vi "Lab Panel V5.26.vi"() -> ()   [LabVIEW 2017] (continued)
                    n1483 = Unbundle(w2774) -> ("T-RISE mins"=w2773:dbl)  [unwired: 4 out]
                    n1484 = Greater Or Equal?(x=w2776, y=w2775) -> (x >= y?=w2777:bool)
                    n1485 = case shown="True" w2777 {
                      tunnel: w2773 -> [w2780 _]
                      tunnel: w2772 -> [w2779 _]
                      tunnel: w2771 -> [w2778 _]
                      frame True {
                        n1486 = stacked-sequence {
                          tunnel: w2780 -> [w2783 _]
                          tunnel: w2779 -> [_ w2788]
                          tunnel: w2778 -> [w2781 _]
                          frame #0 {
                            n1487 = Build Array("T-RISE") -> (w2785:string[])
                            n1488 = Build Array(w2783) -> (w2784:dbl[])
                            n1489 = TDMS Write(0:w2781, 5:"TEST PASS", 7:w2785, 9:w2784) -> (15:w2787:errorcluster)  [unwired: 2 in, 3 out]
                            n1490 = local write "data file error"(w2787) -> ()
                          }
                          frame #1 {
                            n1491 = Bundle(cluster=w2788, "STATUS"="T-RISE PASS") -> (w2790:T4)  [unwired: 2 in]
                            n1492 = local write "RESULT LAB04-2"(TRUE) -> ()
                            n1493 = local write "DISP LAB04-2"(w2790) -> ()
                          }
                        }
                      }
                      frame False {
                      }
                    }
                  }
                }
              }
              frame #8 {
                # "LAB05-1"
                n1494 = Equal?(x=w2793, y=2) -> (x = y?=w2796:bool)
                n1495 = local read "DISP LAB05-1"() -> (w2798:T4)
                n1496 = Unbundle(w2798) -> ("STATUS"=w2799:string)  [unwired: 2 out]
                n1497 = Equal?(x=w2799, y="RUN") -> (x = y?=w2795:bool)
                n1498 = And(x=w2795, y=w2796) -> (x .and. y?=w2794:bool)
                n1499 = case shown="True" w2794 {
                  tunnel: w2798 -> [_ w2802]
                  tunnel: w2792 -> [_ w2805]
                  frame False {
                  }
                  frame True {
                    n1500 = local read "SET LAB05-1"() -> (w2804:T5)
                    n1501 = local read "TDMS LAB05-1"() -> (w2801:refnum<k34>)
                    n1502 = Unbundle(w2802) -> ("CYCLE"=w2806:dbl)  [unwired: 2 out]
                    n1503 = Unbundle(w2804) -> ("T-RISE mins"=w2803:dbl)  [unwired: 4 out]
                    n1504 = Greater Or Equal?(x=w2806, y=w2805) -> (x >= y?=w2807:bool)
                    n1505 = case shown="True" w2807 {
                      tunnel: w2803 -> [w2810 _]
                      tunnel: w2802 -> [w2809 _]
                      tunnel: w2801 -> [w2808 _]
                      frame True {
                        n1506 = stacked-sequence {
                          tunnel: w2810 -> [w2813 _]
                          tunnel: w2809 -> [_ w2818]
                          tunnel: w2808 -> [w2811 _]
                          frame #0 {
                            n1507 = Build Array("T-RISE") -> (w2815:string[])
                            n1508 = Build Array(w2813) -> (w2814:dbl[])
                            n1509 = TDMS Write(0:w2811, 5:"TEST PASS", 7:w2815, 9:w2814) -> (15:w2817:errorcluster)  [unwired: 2 in, 3 out]
                            n1510 = local write "data file error"(w2817) -> ()
                          }
                          frame #1 {
                            n1511 = Bundle(cluster=w2818, "STATUS"="T-RISE PASS") -> (w2820:T4)  [unwired: 2 in]
                            n1512 = local write "RESULT LAB05-1"(TRUE) -> ()
                            n1513 = local write "DISP LAB05-1"(w2820) -> ()
                          }
                        }
                      }
                      frame False {
                      }
                    }
                  }
                }
              }
              frame #9 {
                # "LAB05-2"
                n1514 = Equal?(x=w2823, y=2) -> (x = y?=w2826:bool)
                n1515 = local read "DISP LAB05-2"() -> (w2828:T4)
                n1516 = Unbundle(w2828) -> ("STATUS"=w2829:string)  [unwired: 2 out]
                n1517 = Equal?(x=w2829, y="RUN") -> (x = y?=w2825:bool)
                n1518 = And(x=w2825, y=w2826) -> (x .and. y?=w2824:bool)
                n1519 = case shown="True" w2824 {
                  tunnel: w2828 -> [_ w2832]
                  tunnel: w2822 -> [_ w2835]
                  frame False {
                  }
                  frame True {
                    n1520 = local read "SET LAB05-2"() -> (w2834:T5)
                    n1521 = local read "TDMS LAB05-2"() -> (w2831:refnum<k34>)
                    n1522 = Unbundle(w2832) -> ("CYCLE"=w2836:dbl)  [unwired: 2 out]
                    n1523 = Unbundle(w2834) -> ("T-RISE mins"=w2833:dbl)  [unwired: 4 out]
                    n1524 = Greater Or Equal?(x=w2836, y=w2835) -> (x >= y?=w2837:bool)
                    n1525 = case shown="True" w2837 {
                      tunnel: w2833 -> [w2840 _]
                      tunnel: w2832 -> [w2839 _]
                      tunnel: w2831 -> [w2838 _]
                      frame True {
                        n1526 = stacked-sequence {
                          tunnel: w2840 -> [w2843 _]
                          tunnel: w2839 -> [_ w2848]
                          tunnel: w2838 -> [w2841 _]
                          frame #0 {
                            n1527 = Build Array("T-RISE") -> (w2845:string[])
                            n1528 = Build Array(w2843) -> (w2844:dbl[])
                            n1529 = TDMS Write(0:w2841, 5:"TEST PASS", 7:w2845, 9:w2844) -> (15:w2847:errorcluster)  [unwired: 2 in, 3 out]
                            n1530 = local write "data file error"(w2847) -> ()
                          }
                          frame #1 {
                            n1531 = Bundle(cluster=w2848, "STATUS"="T-RISE PASS") -> (w2850:T4)  [unwired: 2 in]
                            n1532 = local write "RESULT LAB05-2"(TRUE) -> ()
                            n1533 = local write "DISP LAB05-2"(w2850) -> ()
                          }
                        }
                      }
                      frame False {
                      }
                    }
                  }
                }
              }
            }
          }
          frame #7 {
            # "end test & close test files"
            n1534 = local read "MAIL SETTINGS"() -> (w2856:T7)
            n1535 = Unbundle(w2856) -> ("OUT SERVER ADDRESS"=w2855:string, "FROM ACCOUNT"=w2854:string)  [unwired: 5 out]
            n1536 = stacked-sequence {
              tunnel: w2866 -> [_ _ _ _ _ _ _ _ _ _]
              tunnel: w2867 -> [_ _ _ _ _ _ _ _ _ _]
              tunnel: w2865 -> [_ _ _ _ _ _ _ _ _ _]
              tunnel: w2864 -> [_ _ _ _ _ _ _ _ _ _]
              tunnel: w2863 -> [_ _ _ _ _ _ _ _ _ _]
              tunnel: w2862 -> [_ _ _ _ _ _ _ _ _ _]
              tunnel: w2861 -> [_ _ _ _ _ _ _ _ _ _]
              tunnel: w2860 -> [_ _ _ _ _ _ _ _ _ _]
              tunnel: w2859 -> [_ _ _ _ _ _ _ _ _ _]
              tunnel: w2858 -> [_ _ _ _ _ _ _ _ _ _]
              tunnel: w2855 -> [w2871 w2923 w2971 w3018 w3065 w3112 w3159 w3206 w3253 w3300]
              tunnel: w2854 -> [w2870 w2922 w2970 w3017 w3064 w3111 w3158 w3205 w3252 w3299]
              tunnel: "Mail Test File To:" -> [w2869 w2921 w2969 w3016 w3063 w3110 w3157 w3204 w3251 w3298]
              tunnel: "Mail Test Fail" -> [w2868 w2920 w2968 w3015 w3062 w3109 w3156 w3203 w3250 w3297]
              frame #0 {
                # "LAB01-1"
                n1537 = local read "DISP LAB01-1"() -> (w2875:T4)
                n1538 = local read "run lab01-1"() -> (w2872:bool)
                n1539 = local read "TDMS LAB01-1"() -> (w2873:refnum<k34>)
                n1540 = Unbundle(w2875) -> ("CYCLE"=w2876:dbl, "STATUS"=w2874:string)  [unwired: 1 out]
                n1541 = case shown="True" w2872 {
                  tunnel: w2876 -> [_ w2882]
                  tunnel: w2875 -> [_ w2884]
                  tunnel: w2874 -> [_ w2881]
                  tunnel: w2873 -> [_ w2883]
                  tunnel: w2871 -> [_ w2880]
                  tunnel: w2870 -> [_ w2879]
                  tunnel: w2869 -> [_ w2878]
                  tunnel: w2868 -> [_ w2877]
                  frame False {
                  }
                  frame True {
                    n1542 = Not Equal?(x=w2881, y="RUN") -> (x != y?=w2885:bool)
                    n1543 = Greater?(x=w2882, y=2.0) -> (0:w2887:bool)
                    n1544 = And(x=w2887, y=w2885) -> (x .and. y?=w2886:bool)
                    n1545 = case shown="True" w2886 {
                      tunnel: w2884 -> [_ w2897]
                      tunnel: w2883 -> [_ w2896]
                      tunnel: w2882 -> [_ w2895]
                      tunnel: w2881 -> [_ w2894]
                      tunnel: w2880 -> [_ w2893]
                      tunnel: w2879 -> [_ w2892]
                      tunnel: w2878 -> [_ w2891]
                      tunnel: w2877 -> [_ w2890]
                      frame False {
                      }
                      frame True {
                        n1546 = stacked-sequence {
                          tunnel: w2897 -> [w2901 _ _]
                          tunnel: w2896 -> [_ w2903 _]
                          tunnel: w2895 -> [_ _ _]
                          tunnel: w2894 -> [_ _ w2909]
                          tunnel: w2893 -> [_ _ w2908]
                          tunnel: w2892 -> [_ _ w2907]
                          tunnel: w2891 -> [_ _ w2906]
                          tunnel: w2890 -> [_ _ w2905]
                          frame #0 {
                            w2898 = FALSE
                            n1547 = local write "mail control"("END") -> ()
                            n1548 = Bundle(cluster=w2901) -> (w2900:T4)  [unwired: 3 in]
                            n1549 = local write "DISP LAB01-1"(w2900) -> ()
                            n1550 = local write "O/I  LAB01-1"(w2898) -> ()
                            n1551 = local write "run lab01-1"(w2898) -> ()
                            n1552 = local write "RUN LAB01-1"(w2898) -> ()
                          }
                          frame #1 {
                            n1553 = TDMS Close(11:w2903) -> (0:w2902:errorcluster)  [unwired: 1 in, 1 out]
                            n1554 = local write "data file error"(w2902) -> ()
                          }
                          frame #2 {
                            n1555 = stacked-sequence {
                              tunnel: "LAB01-1" -> [w2911 w2913 _]
                              tunnel: w2909 -> [_ w2919 _]
                              tunnel: w2908 -> [_ w2918 _]
                              tunnel: w2907 -> [_ w2917 _]
                              tunnel: w2906 -> [_ w2916 _]
                              tunnel: w2905 -> [_ w2915 _]
                              frame #0 {
                                n1556 = call "sub vi - defrag tdms v1.vi"("panel id"=w2911) -> ("error out"=w2910:errorcluster)  [unwired: 10 in]
                                n1557 = local write "data file error"(w2910) -> ()
                              }
                              frame #1 {
                                n1558 = Bundle("STATUS"=w2919, "OUT SERVER ADDRESS"=w2918, "FROM ACCOUNT"=w2917, "Mail Test File To:"=w2916, "Mail Test Fail"=w2915) -> (w2912:T26)  [unwired: 1 in]
                                n1559 = call "Save data file (pass-fail) v5.vi"("Input Cluster"=w2912, "panel id"=w2913) -> ("network file save error"=w2914:errorcluster)  [unwired: 8 in, 1 out]
                                n1560 = local write "data file error"(w2914) -> ()
                              }
                              frame #2 {
                              }
                            }
                          }
                        }
                      }
                    }
                  }
                }
              }
              frame #1 {
                # "LAB01-2"
                n1561 = local read "run lab01-2"() -> (w2924:bool)
                n1562 = case shown="True" w2924 {
                  tunnel: w2923 -> [_ w2928]
                  tunnel: w2922 -> [_ w2927]
                  tunnel: w2921 -> [_ w2926]
                  tunnel: w2920 -> [_ w2925]
                  frame False {
                  }
                  frame True {
                    n1563 = local read "DISP LAB01-2"() -> (w2936:T4)
                    n1564 = local read "TDMS LAB01-2"() -> (w2935:refnum<k34>)
                    n1565 = Unbundle(w2936) -> ("CYCLE"=w2930:dbl, "STATUS"=w2929:string)  [unwired: 1 out]
                    n1566 = Not Equal?(x=w2929, y="RUN") -> (x != y?=w2932:bool)
                    n1567 = Greater?(x=w2930, y=2.0) -> (0:w2933:bool)
                    n1568 = And(x=w2933, y=w2932) -> (x .and. y?=w2931:bool)
                    n1569 = case shown="True" w2931 {
                      tunnel: w2936 -> [_ w2945]
                      tunnel: w2935 -> [_ w2944]
                      tunnel: w2930 -> [_ w2943]
                      tunnel: w2929 -> [_ w2942]
                      tunnel: w2928 -> [_ w2941]
                      tunnel: w2927 -> [_ w2940]
                      tunnel: w2926 -> [_ w2939]
                      tunnel: w2925 -> [_ w2938]
                      frame False {
                      }
                      frame True {
                        n1570 = stacked-sequence {
                          tunnel: w2945 -> [w2948 _ _]
                          tunnel: w2944 -> [_ w2950 _]
                          tunnel: w2943 -> [_ _ _]
                          tunnel: w2942 -> [_ _ w2956]
                          tunnel: w2941 -> [_ _ w2955]
                          tunnel: w2940 -> [_ _ w2954]
                          tunnel: w2939 -> [_ _ w2953]
                          tunnel: w2938 -> [_ _ w2952]
                          frame #0 {
                            w2946 = FALSE
                            n1571 = local write "mail control"("END") -> ()
                            n1572 = Bundle(cluster=w2948) -> (w2949:T4)  [unwired: 3 in]
                            n1573 = local write "RUN LAB01-2"(w2946) -> ()
                            n1574 = local write "run lab01-2"(w2946) -> ()
                            n1575 = local write "O/I  LAB01-2"(w2946) -> ()
                            n1576 = local write "DISP LAB01-2"(w2949) -> ()
                          }
                          frame #1 {
                            n1577 = TDMS Close(11:w2950) -> (0:w2951:errorcluster)  [unwired: 1 in, 1 out]
                            n1578 = local write "data file error"(w2951) -> ()
                          }
                          frame #2 {
                            n1579 = stacked-sequence {
                              tunnel: "LAB01-2" -> [w2959 w2960]
                              tunnel: w2956 -> [_ w2965]
                              tunnel: w2955 -> [_ w2964]
                              tunnel: w2954 -> [_ w2963]
                              tunnel: w2953 -> [_ w2962]
                              tunnel: w2952 -> [_ w2961]
                              frame #0 {
                                n1580 = call "sub vi - defrag tdms v1.vi"("panel id"=w2959) -> ("error out"=w2958:errorcluster)  [unwired: 10 in]
                                n1581 = local write "data file error"(w2958) -> ()
                              }
                              frame #1 {
                                n1582 = Bundle("STATUS"=w2965, "OUT SERVER ADDRESS"=w2964, "FROM ACCOUNT"=w2963, "Mail Test File To:"=w2962, "Mail Test Fail"=w2961) -> (w2967:T26)  [unwired: 1 in]
                                n1583 = call "Save data file (pass-fail) v5.vi"("Input Cluster"=w2967, "panel id"=w2960) -> ("network file save error"=w2966:errorcluster)  [unwired: 8 in, 1 out]
                                n1584 = local write "data file error"(w2966) -> ()
                              }
                            }
                          }
                        }
                      }
                    }
                  }
                }
              }
              frame #2 {
                # "LAB02-1"
                n1585 = local read "run lab02-1"() -> (w2972:bool)
                n1586 = case shown="True" w2972 {
                  tunnel: w2971 -> [_ w2976]
                  tunnel: w2970 -> [_ w2975]
                  tunnel: w2969 -> [_ w2974]
                  tunnel: w2968 -> [_ w2973]
                  frame False {
                  }
                  frame True {
                    n1587 = local read "DISP LAB02-1"() -> (w2984:T4)
                    n1588 = Unbundle(w2984) -> ("CYCLE"=w2980:dbl, "STATUS"=w2977:string)  [unwired: 1 out]
                    n1589 = local read "TDMS LAB02-1"() -> (w2983:refnum<k34>)
                    n1590 = Not Equal?(x=w2977, y="RUN") -> (x != y?=w2979:bool)
                    n1591 = Greater?(x=w2980, y=2.0) -> (0:w2981:bool)
                    n1592 = And(x=w2981, y=w2979) -> (x .and. y?=w2978:bool)
                    n1593 = case shown="True" w2978 {
                      tunnel: w2984 -> [_ w2992]
                      tunnel: w2983 -> [_ w2991]
                      tunnel: w2977 -> [_ w2990]
                      tunnel: w2976 -> [_ w2989]
                      tunnel: w2975 -> [_ w2988]
                      tunnel: w2974 -> [_ w2987]
                      tunnel: w2973 -> [_ w2986]
                      frame False {
                      }
                      frame True {
                        n1594 = stacked-sequence {
                          tunnel: w2992 -> [w2995 _ _]
                          tunnel: w2991 -> [_ w2997 _]
                          tunnel: w2990 -> [_ _ w3003]
                          tunnel: w2989 -> [_ _ w3002]
                          tunnel: w2988 -> [_ _ w3001]
                          tunnel: w2987 -> [_ _ w3000]
                          tunnel: w2986 -> [_ _ w2999]
                          frame #0 {
                            w2993 = FALSE
                            n1595 = local write "mail control"("END") -> ()
                            n1596 = Bundle(cluster=w2995) -> (w2996:T4)  [unwired: 3 in]
                            n1597 = local write "O/I  LAB02-1"(w2993) -> ()
                            n1598 = local write "RUN LAB02-1"(w2993) -> ()
                            n1599 = local write "run lab02-1"(w2993) -> ()
                            n1600 = local write "DISP LAB02-1"(w2996) -> ()
                          }
                          frame #1 {
                            n1601 = TDMS Close(11:w2997) -> (0:w2998:errorcluster)  [unwired: 1 in, 1 out]
                            n1602 = local write "data file error"(w2998) -> ()
                          }
                          frame #2 {
                            n1603 = stacked-sequence {
                              tunnel: "LAB02-1" -> [w3006 w3013]
                              tunnel: w3003 -> [_ w3011]
                              tunnel: w3002 -> [_ w3010]
                              tunnel: w3001 -> [_ w3009]
                              tunnel: w3000 -> [_ w3008]
                              tunnel: w2999 -> [_ w3007]
                              frame #0 {
                                n1604 = call "sub vi - defrag tdms v1.vi"("panel id"=w3006) -> ("error out"=w3005:errorcluster)  [unwired: 10 in]
                                n1605 = local write "data file error"(w3005) -> ()
                              }
                              frame #1 {
                                n1606 = Bundle("STATUS"=w3011, "OUT SERVER ADDRESS"=w3010, "FROM ACCOUNT"=w3009, "Mail Test File To:"=w3008, "Mail Test Fail"=w3007) -> (w3012:T26)  [unwired: 1 in]
                                n1607 = call "Save data file (pass-fail) v5.vi"("Input Cluster"=w3012, "panel id"=w3013) -> ("network file save error"=w3014:errorcluster)  [unwired: 8 in, 1 out]
                                n1608 = local write "data file error"(w3014) -> ()
                              }
                            }
                          }
                        }
                      }
                    }
                  }
                }
              }
              frame #3 {
                # "LAB02-2"
                n1609 = local read "run lab02-2"() -> (w3019:bool)
                n1610 = case shown="True" w3019 {
                  tunnel: w3018 -> [_ w3023]
                  tunnel: w3017 -> [_ w3022]
                  tunnel: w3016 -> [_ w3021]
                  tunnel: w3015 -> [_ w3020]
                  frame False {
                  }
                  frame True {
                    n1611 = local read "DISP LAB02-2"() -> (w3031:T4)
                    n1612 = local read "TDMS LAB02-2"() -> (w3030:refnum<k34>)
                    n1613 = Unbundle(w3031) -> ("CYCLE"=w3027:dbl, "STATUS"=w3024:string)  [unwired: 1 out]
                    n1614 = Not Equal?(x=w3024, y="RUN") -> (x != y?=w3026:bool)
                    n1615 = Greater?(x=w3027, y=2.0) -> (0:w3028:bool)
                    n1616 = And(x=w3028, y=w3026) -> (x .and. y?=w3025:bool)
                    n1617 = case shown="True" w3025 {
                      tunnel: w3031 -> [_ w3039]
                      tunnel: w3030 -> [_ w3038]
                      tunnel: w3024 -> [_ w3037]
                      tunnel: w3023 -> [_ w3036]
                      tunnel: w3022 -> [_ w3035]
                      tunnel: w3021 -> [_ w3034]
                      tunnel: w3020 -> [_ w3033]
                      frame False {
                      }
                      frame True {
                        n1618 = stacked-sequence {
                          tunnel: w3039 -> [w3042 _ _]
                          tunnel: w3038 -> [_ w3044 _]
                          tunnel: w3037 -> [_ _ w3050]
                          tunnel: w3036 -> [_ _ w3049]
                          tunnel: w3035 -> [_ _ w3048]
                          tunnel: w3034 -> [_ _ w3047]
                          tunnel: w3033 -> [_ _ w3046]
                          frame #0 {
                            w3040 = FALSE
                            n1619 = local write "mail control"("END") -> ()
                            n1620 = Bundle(cluster=w3042) -> (w3043:T4)  [unwired: 3 in]
                            n1621 = local write "O/I  LAB02-2"(w3040) -> ()
                            n1622 = local write "run lab02-2"(w3040) -> ()
                            n1623 = local write "RUN LAB02-2"(w3040) -> ()
                            n1624 = local write "DISP LAB02-2"(w3043) -> ()
                          }
                          frame #1 {
                            n1625 = TDMS Close(11:w3044) -> (0:w3045:errorcluster)  [unwired: 1 in, 1 out]
                            n1626 = local write "data file error"(w3045) -> ()
                          }
                          frame #2 {
                            n1627 = stacked-sequence {
                              tunnel: "LAB02-2" -> [w3053 w3059]
                              tunnel: w3050 -> [_ w3058]
                              tunnel: w3049 -> [_ w3057]
                              tunnel: w3048 -> [_ w3056]
                              tunnel: w3047 -> [_ w3055]
                              tunnel: w3046 -> [_ w3054]
                              frame #0 {
                                n1628 = call "sub vi - defrag tdms v1.vi"("panel id"=w3053) -> ("error out"=w3052:errorcluster)  [unwired: 10 in]
                                n1629 = local write "data file error"(w3052) -> ()
                              }
                              frame #1 {
                                n1630 = Bundle("STATUS"=w3058, "OUT SERVER ADDRESS"=w3057, "FROM ACCOUNT"=w3056, "Mail Test File To:"=w3055, "Mail Test Fail"=w3054) -> (w3061:T26)  [unwired: 1 in]
                                n1631 = call "Save data file (pass-fail) v5.vi"("Input Cluster"=w3061, "panel id"=w3059) -> ("network file save error"=w3060:errorcluster)  [unwired: 8 in, 1 out]
                                n1632 = local write "data file error"(w3060) -> ()
                              }
                            }
                          }
                        }
                      }
                    }
                  }
                }
              }
              frame #4 {
                # "LAB03-1"
                n1633 = local read "run lab03-1"() -> (w3066:bool)
                n1634 = case shown="True" w3066 {
                  tunnel: w3065 -> [_ w3070]
                  tunnel: w3064 -> [_ w3069]
                  tunnel: w3063 -> [_ w3068]
                  tunnel: w3062 -> [_ w3067]
                  frame False {
                  }
                  frame True {
                    n1635 = local read "DISP LAB03-1"() -> (w3078:T4)
                    n1636 = local read "TDMS LAB03-1"() -> (w3077:refnum<k34>)
                    n1637 = Unbundle(w3078) -> ("CYCLE"=w3074:dbl, "STATUS"=w3071:string)  [unwired: 1 out]
                    n1638 = Not Equal?(x=w3071, y="RUN") -> (x != y?=w3073:bool)
                    n1639 = Greater?(x=w3074, y=2.0) -> (0:w3075:bool)
                    n1640 = And(x=w3075, y=w3073) -> (x .and. y?=w3072:bool)
                    n1641 = case shown="True" w3072 {
                      tunnel: w3078 -> [_ w3086]
                      tunnel: w3077 -> [_ w3085]
                      tunnel: w3071 -> [_ w3084]
                      tunnel: w3070 -> [_ w3083]
                      tunnel: w3069 -> [_ w3082]
                      tunnel: w3068 -> [_ w3081]
                      tunnel: w3067 -> [_ w3080]
                      frame False {
                      }
                      frame True {
                        n1642 = stacked-sequence {
                          tunnel: w3086 -> [w3089 _ _]
                          tunnel: w3085 -> [_ w3091 _]
                          tunnel: w3084 -> [_ _ w3097]
                          tunnel: w3083 -> [_ _ w3096]
                          tunnel: w3082 -> [_ _ w3095]
                          tunnel: w3081 -> [_ _ w3094]
                          tunnel: w3080 -> [_ _ w3093]
                          frame #0 {
                            w3087 = FALSE
                            n1643 = local write "mail control"("END") -> ()
                            n1644 = Bundle(cluster=w3089) -> (w3090:T4)  [unwired: 3 in]
                            n1645 = local write "O/I  LAB03-1"(w3087) -> ()
                            n1646 = local write "run lab03-1"(w3087) -> ()
                            n1647 = local write "RUN LAB03-1"(w3087) -> ()
                            n1648 = local write "DISP LAB03-1"(w3090) -> ()
                          }
                          frame #1 {
                            n1649 = TDMS Close(11:w3091) -> (0:w3092:errorcluster)  [unwired: 1 in, 1 out]
                            n1650 = local write "data file error"(w3092) -> ()
                          }
                          frame #2 {
                            n1651 = stacked-sequence {
                              tunnel: "LAB03-1" -> [w3100 w3106]
                              tunnel: w3097 -> [_ w3105]
                              tunnel: w3096 -> [_ w3104]
                              tunnel: w3095 -> [_ w3103]
                              tunnel: w3094 -> [_ w3102]
                              tunnel: w3093 -> [_ w3101]
                              frame #0 {
                                n1652 = call "sub vi - defrag tdms v1.vi"("panel id"=w3100) -> ("error out"=w3099:errorcluster)  [unwired: 10 in]
                                n1653 = local write "data file error"(w3099) -> ()
                              }
                              frame #1 {
                                n1654 = Bundle("STATUS"=w3105, "OUT SERVER ADDRESS"=w3104, "FROM ACCOUNT"=w3103, "Mail Test File To:"=w3102, "Mail Test Fail"=w3101) -> (w3108:T26)  [unwired: 1 in]
                                n1655 = call "Save data file (pass-fail) v5.vi"("Input Cluster"=w3108, "panel id"=w3106) -> ("network file save error"=w3107:errorcluster)  [unwired: 8 in, 1 out]
                                n1656 = local write "data file error"(w3107) -> ()
                              }
                            }
                          }
                        }
                      }
                    }
                  }
                }
              }
              frame #5 {
                # "LAB03-2"
                n1657 = local read "run lab03-2"() -> (w3113:bool)
                n1658 = case shown="True" w3113 {
                  tunnel: w3112 -> [_ w3117]
                  tunnel: w3111 -> [_ w3116]
                  tunnel: w3110 -> [_ w3115]
                  tunnel: w3109 -> [_ w3114]
                  frame False {
                  }
                  frame True {
                    n1659 = local read "DISP LAB03-2"() -> (w3125:T4)
                    n1660 = Unbundle(w3125) -> ("CYCLE"=w3121:dbl, "STATUS"=w3118:string)  [unwired: 1 out]
                    n1661 = local read "TDMS LAB03-2"() -> (w3124:refnum<k34>)
                    n1662 = Not Equal?(x=w3118, y="RUN") -> (x != y?=w3120:bool)
                    n1663 = Greater?(x=w3121, y=2.0) -> (0:w3122:bool)
                    n1664 = And(x=w3122, y=w3120) -> (x .and. y?=w3119:bool)
                    n1665 = case shown="True" w3119 {
                      tunnel: w3125 -> [_ w3133]
                      tunnel: w3124 -> [_ w3132]
                      tunnel: w3118 -> [_ w3131]
                      tunnel: w3117 -> [_ w3130]
                      tunnel: w3116 -> [_ w3129]
                      tunnel: w3115 -> [_ w3128]
                      tunnel: w3114 -> [_ w3127]
                      frame False {
                      }
                      frame True {
                        n1666 = stacked-sequence {
                          tunnel: w3133 -> [w3136 _ _]
                          tunnel: w3132 -> [_ w3138 _]
                          tunnel: w3131 -> [_ _ w3144]
                          tunnel: w3130 -> [_ _ w3143]
                          tunnel: w3129 -> [_ _ w3142]
                          tunnel: w3128 -> [_ _ w3141]
                          tunnel: w3127 -> [_ _ w3140]
                          frame #0 {
                            w3134 = FALSE
                            n1667 = local write "mail control"("END") -> ()
                            n1668 = Bundle(cluster=w3136) -> (w3137:T4)  [unwired: 3 in]
                            n1669 = local write "RUN LAB03-2"(w3134) -> ()
                            n1670 = local write "O/I  LAB03-2"(w3134) -> ()
                            n1671 = local write "DISP LAB03-2"(w3137) -> ()
                            n1672 = local write "run lab03-2"(w3134) -> ()
                          }
                          frame #1 {
                            n1673 = TDMS Close(11:w3138) -> (0:w3139:errorcluster)  [unwired: 1 in, 1 out]
                            n1674 = local write "data file error"(w3139) -> ()
                          }
                          frame #2 {
                            n1675 = stacked-sequence {
                              tunnel: "LAB03-2" -> [w3147 w3148]
                              tunnel: w3144 -> [_ w3153]
                              tunnel: w3143 -> [_ w3152]
                              tunnel: w3142 -> [_ w3151]
                              tunnel: w3141 -> [_ w3150]
                              tunnel: w3140 -> [_ w3149]
                              frame #0 {
                                n1676 = call "sub vi - defrag tdms v1.vi"("panel id"=w3147) -> ("error out"=w3146:errorcluster)  [unwired: 10 in]
                                n1677 = local write "data file error"(w3146) -> ()
                              }
                              frame #1 {
                                n1678 = Bundle("STATUS"=w3153, "OUT SERVER ADDRESS"=w3152, "FROM ACCOUNT"=w3151, "Mail Test File To:"=w3150, "Mail Test Fail"=w3149) -> (w3155:T26)  [unwired: 1 in]
                                n1679 = call "Save data file (pass-fail) v5.vi"("Input Cluster"=w3155, "panel id"=w3148) -> ("network file save error"=w3154:errorcluster)  [unwired: 8 in, 1 out]
                                n1680 = local write "data file error"(w3154) -> ()
                              }
                            }
                          }
                        }
                      }
                    }
                  }
                }
              }
              frame #6 {
                # "LAB04-1"
                n1681 = local read "run lab04-1"() -> (w3160:bool)
                n1682 = case shown="True" w3160 {
                  tunnel: w3159 -> [_ w3164]
                  tunnel: w3158 -> [_ w3163]
                  tunnel: w3157 -> [_ w3162]
                  tunnel: w3156 -> [_ w3161]
                  frame False {
                  }
                  frame True {
                    n1683 = local read "DISP LAB04-1"() -> (w3172:T4)
                    n1684 = Unbundle(w3172) -> ("CYCLE"=w3168:dbl, "STATUS"=w3165:string)  [unwired: 1 out]
                    n1685 = local read "TDMS LAB04-1"() -> (w3171:refnum<k34>)
                    n1686 = Not Equal?(x=w3165, y="RUN") -> (x != y?=w3167:bool)
                    n1687 = Greater?(x=w3168, y=2.0) -> (0:w3169:bool)
                    n1688 = And(x=w3169, y=w3167) -> (x .and. y?=w3166:bool)
                    n1689 = case shown="True" w3166 {
                      tunnel: w3172 -> [_ w3180]
                      tunnel: w3171 -> [_ w3179]
                      tunnel: w3165 -> [_ w3178]
                      tunnel: w3164 -> [_ w3177]
                      tunnel: w3163 -> [_ w3176]
                      tunnel: w3162 -> [_ w3175]
                      tunnel: w3161 -> [_ w3174]
                      frame False {
                      }
                      frame True {
                        n1690 = stacked-sequence {
                          tunnel: w3180 -> [w3183 _ _]
                          tunnel: w3179 -> [_ w3185 _]
                          tunnel: w3178 -> [_ _ w3191]
                          tunnel: w3177 -> [_ _ w3190]
                          tunnel: w3176 -> [_ _ w3189]
                          tunnel: w3175 -> [_ _ w3188]
                          tunnel: w3174 -> [_ _ w3187]
                          frame #0 {
                            w3181 = FALSE
                            n1691 = local write "mail control"("END") -> ()
                            n1692 = Bundle(cluster=w3183) -> (w3184:T4)  [unwired: 3 in]
                            n1693 = local write "RUN LAB04-1"(w3181) -> ()
                            n1694 = local write "O/I  LAB04-1"(w3181) -> ()
                            n1695 = local write "run lab04-1"(w3181) -> ()
                            n1696 = local write "DISP LAB04-1"(w3184) -> ()
                          }
                          frame #1 {
                            n1697 = TDMS Close(11:w3185) -> (0:w3186:errorcluster)  [unwired: 1 in, 1 out]
                            n1698 = local write "data file error"(w3186) -> ()
                          }
                          frame #2 {
                            n1699 = stacked-sequence {
                              tunnel: "LAB04-1" -> [w3194 w3195]
                              tunnel: w3191 -> [_ w3200]
                              tunnel: w3190 -> [_ w3199]
                              tunnel: w3189 -> [_ w3198]
                              tunnel: w3188 -> [_ w3197]
                              tunnel: w3187 -> [_ w3196]
                              frame #0 {
                                n1700 = call "sub vi - defrag tdms v1.vi"("panel id"=w3194) -> ("error out"=w3193:errorcluster)  [unwired: 10 in]
                                n1701 = local write "data file error"(w3193) -> ()
                              }
                              frame #1 {
                                n1702 = Bundle("STATUS"=w3200, "OUT SERVER ADDRESS"=w3199, "FROM ACCOUNT"=w3198, "Mail Test File To:"=w3197, "Mail Test Fail"=w3196) -> (w3202:T26)  [unwired: 1 in]
                                n1703 = call "Save data file (pass-fail) v5.vi"("Input Cluster"=w3202, "panel id"=w3195) -> ("network file save error"=w3201:errorcluster)  [unwired: 8 in, 1 out]
                                n1704 = local write "data file error"(w3201) -> ()
                              }
                            }
                          }
                        }
                      }
                    }
                  }
                }
              }
              frame #7 {
                # "LAB04-2"
                n1705 = local read "run lab04-2"() -> (w3207:bool)
                n1706 = case shown="True" w3207 {
                  tunnel: w3206 -> [_ w3211]
                  tunnel: w3205 -> [_ w3210]
                  tunnel: w3204 -> [_ w3209]
                  tunnel: w3203 -> [_ w3208]
                  frame False {
                  }
                  frame True {
                    n1707 = local read "DISP LAB04-2"() -> (w3219:T4)
                    n1708 = Unbundle(w3219) -> ("CYCLE"=w3215:dbl, "STATUS"=w3212:string)  [unwired: 1 out]
                    n1709 = Not Equal?(x=w3212, y="RUN") -> (x != y?=w3214:bool)
                    n1710 = local read "TDMS LAB04-2"() -> (w3218:refnum<k34>)
                    n1711 = Greater?(x=w3215, y=2.0) -> (0:w3216:bool)
                    n1712 = And(x=w3216, y=w3214) -> (x .and. y?=w3213:bool)
                    n1713 = case shown="True" w3213 {
                      tunnel: w3219 -> [_ w3227]
                      tunnel: w3218 -> [_ w3226]
                      tunnel: w3212 -> [_ w3225]
                      tunnel: w3211 -> [_ w3224]
                      tunnel: w3210 -> [_ w3223]
                      tunnel: w3209 -> [_ w3222]
                      tunnel: w3208 -> [_ w3221]
                      frame False {
                      }
                      frame True {
                        n1714 = stacked-sequence {
                          tunnel: w3227 -> [w3230 _ _]
                          tunnel: w3226 -> [_ w3232 _]
                          tunnel: w3225 -> [_ _ w3238]
                          tunnel: w3224 -> [_ _ w3237]
                          tunnel: w3223 -> [_ _ w3236]
                          tunnel: w3222 -> [_ _ w3235]
                          tunnel: w3221 -> [_ _ w3234]
                          frame #0 {
                            w3228 = FALSE
                            n1715 = local write "mail control"("END") -> ()
                            n1716 = Bundle(cluster=w3230) -> (w3231:T4)  [unwired: 3 in]
                            n1717 = local write "O/I  LAB04-2"(w3228) -> ()
                            n1718 = local write "RUN LAB04-2"(w3228) -> ()
                            n1719 = local write "run lab04-2"(w3228) -> ()
                            n1720 = local write "DISP LAB04-2"(w3231) -> ()
                          }
                          frame #1 {
                            n1721 = TDMS Close(11:w3232) -> (0:w3233:errorcluster)  [unwired: 1 in, 1 out]
                            n1722 = local write "data file error"(w3233) -> ()
                          }
                          frame #2 {
                            n1723 = stacked-sequence {
                              tunnel: "LAB04-2" -> [w3241 w3242]
                              tunnel: w3238 -> [_ w3247]
                              tunnel: w3237 -> [_ w3246]
                              tunnel: w3236 -> [_ w3245]
                              tunnel: w3235 -> [_ w3244]
                              tunnel: w3234 -> [_ w3243]
                              frame #0 {
                                n1724 = call "sub vi - defrag tdms v1.vi"("panel id"=w3241) -> ("error out"=w3240:errorcluster)  [unwired: 10 in]
                                n1725 = local write "data file error"(w3240) -> ()
                              }
                              frame #1 {
                                n1726 = Bundle("STATUS"=w3247, "OUT SERVER ADDRESS"=w3246, "FROM ACCOUNT"=w3245, "Mail Test File To:"=w3244, "Mail Test Fail"=w3243) -> (w3249:T26)  [unwired: 1 in]
                                n1727 = call "Save data file (pass-fail) v5.vi"("Input Cluster"=w3249, "panel id"=w3242) -> ("network file save error"=w3248:errorcluster)  [unwired: 8 in, 1 out]
                                n1728 = local write "data file error"(w3248) -> ()
                              }
                            }
                          }
                        }
                      }
                    }
                  }
                }
              }
              frame #8 {
                # "LAB05-1"
                n1729 = local read "run lab05-1"() -> (w3254:bool)
                n1730 = case shown="True" w3254 {
                  tunnel: w3253 -> [_ w3258]
                  tunnel: w3252 -> [_ w3257]
                  tunnel: w3251 -> [_ w3256]
                  tunnel: w3250 -> [_ w3255]
                  frame False {
                  }
                  frame True {
                    n1731 = local read "DISP LAB05-1"() -> (w3266:T4)
                    n1732 = Unbundle(w3266) -> ("CYCLE"=w3262:dbl, "STATUS"=w3259:string)  [unwired: 1 out]
                    n1733 = Not Equal?(x=w3259, y="RUN") -> (x != y?=w3261:bool)
                    n1734 = local read "TDMS LAB05-1"() -> (w3265:refnum<k34>)
                    n1735 = Greater?(x=w3262, y=2.0) -> (0:w3263:bool)
                    n1736 = And(x=w3263, y=w3261) -> (x .and. y?=w3260:bool)
                    n1737 = case shown="True" w3260 {
                      tunnel: w3266 -> [_ w3274]
                      tunnel: w3265 -> [_ w3273]
                      tunnel: w3259 -> [_ w3272]
                      tunnel: w3258 -> [_ w3271]
                      tunnel: w3257 -> [_ w3270]
                      tunnel: w3256 -> [_ w3269]
                      tunnel: w3255 -> [_ w3268]
                      frame False {
                      }
                      frame True {
                        n1738 = stacked-sequence {
                          tunnel: w3274 -> [w3277 _ _]
                          tunnel: w3273 -> [_ w3279 _]
                          tunnel: w3272 -> [_ _ w3285]
                          tunnel: w3271 -> [_ _ w3284]
                          tunnel: w3270 -> [_ _ w3283]
                          tunnel: w3269 -> [_ _ w3282]
                          tunnel: w3268 -> [_ _ w3281]
                          frame #0 {
                            w3275 = FALSE
                            n1739 = local write "mail control"("END") -> ()
                            n1740 = Bundle(cluster=w3277) -> (w3278:T4)  [unwired: 3 in]
                            n1741 = local write "O/I  LAB05-1"(w3275) -> ()
                            n1742 = local write "RUN LAB05-1"(w3275) -> ()
                            n1743 = local write "run lab05-1"(w3275) -> ()
                            n1744 = local write "DISP LAB05-1"(w3278) -> ()
                          }
                          frame #1 {
                            n1745 = TDMS Close(11:w3279) -> (0:w3280:errorcluster)  [unwired: 1 in, 1 out]
                            n1746 = local write "data file error"(w3280) -> ()
                          }
                          frame #2 {
                            n1747 = stacked-sequence {
                              tunnel: "LAB05-1" -> [w3288 w3294]
                              tunnel: w3285 -> [_ w3293]
                              tunnel: w3284 -> [_ w3292]
                              tunnel: w3283 -> [_ w3291]
                              tunnel: w3282 -> [_ w3290]
                              tunnel: w3281 -> [_ w3289]
                              frame #0 {
                                n1748 = call "sub vi - defrag tdms v1.vi"("panel id"=w3288) -> ("error out"=w3287:errorcluster)  [unwired: 10 in]
                                n1749 = local write "data file error"(w3287) -> ()
                              }
                              frame #1 {
                                n1750 = Bundle("STATUS"=w3293, "OUT SERVER ADDRESS"=w3292, "FROM ACCOUNT"=w3291, "Mail Test File To:"=w3290, "Mail Test Fail"=w3289) -> (w3296:T26)  [unwired: 1 in]
                                n1751 = call "Save data file (pass-fail) v5.vi"("Input Cluster"=w3296, "panel id"=w3294) -> ("network file save error"=w3295:errorcluster)  [unwired: 8 in, 1 out]
                                n1752 = local write "data file error"(w3295) -> ()
                              }
                            }
                          }
                        }
                      }
                    }
                  }
                }
              }
              frame #9 {
                # "LAB05-2"
                n1753 = local read "run lab05-2"() -> (w3301:bool)
                n1754 = case shown="True" w3301 {
                  tunnel: w3300 -> [_ w3305]
                  tunnel: w3299 -> [_ w3304]
                  tunnel: w3298 -> [_ w3303]
                  tunnel: w3297 -> [_ w3302]
                  frame False {
                  }
                  frame True {
                    n1755 = local read "DISP LAB05-2"() -> (w3313:T4)
                    n1756 = Unbundle(w3313) -> ("CYCLE"=w3309:dbl, "STATUS"=w3306:string)  [unwired: 1 out]
                    n1757 = Not Equal?(x=w3306, y="RUN") -> (x != y?=w3308:bool)
                    n1758 = local read "TDMS LAB05-2"() -> (w3312:refnum<k34>)
                    n1759 = Greater?(x=w3309, y=2.0) -> (0:w3310:bool)
                    n1760 = And(x=w3310, y=w3308) -> (x .and. y?=w3307:bool)
                    n1761 = case shown="True" w3307 {
                      tunnel: w3313 -> [_ w3321]
                      tunnel: w3312 -> [_ w3320]
                      tunnel: w3306 -> [_ w3319]
                      tunnel: w3305 -> [_ w3318]
                      tunnel: w3304 -> [_ w3317]
                      tunnel: w3303 -> [_ w3316]
                      tunnel: w3302 -> [_ w3315]
                      frame False {
                      }
                      frame True {
                        n1762 = stacked-sequence {
                          tunnel: w3321 -> [w3324 _ _]
                          tunnel: w3320 -> [_ w3326 _]
                          tunnel: w3319 -> [_ _ w3332]
                          tunnel: w3318 -> [_ _ w3331]
                          tunnel: w3317 -> [_ _ w3330]
                          tunnel: w3316 -> [_ _ w3329]
                          tunnel: w3315 -> [_ _ w3328]
                          frame #0 {
                            w3322 = FALSE
                            n1763 = local write "mail control"("END") -> ()
                            n1764 = Bundle(cluster=w3324) -> (w3325:T4)  [unwired: 3 in]
                            n1765 = local write "RUN LAB05-2"(w3322) -> ()
                            n1766 = local write "O/I  LAB05-2"(w3322) -> ()
                            n1767 = local write "run lab05-2"(w3322) -> ()
                            n1768 = local write "DISP LAB05-2"(w3325) -> ()
                          }
                          frame #1 {
                            n1769 = TDMS Close(11:w3326) -> (0:w3327:errorcluster)  [unwired: 1 in, 1 out]
                            n1770 = local write "data file error"(w3327) -> ()
                          }
                          frame #2 {
                            n1771 = stacked-sequence {
                              tunnel: "LAB05-2" -> [w3335 w3341]
                              tunnel: w3332 -> [_ w3340]
                              tunnel: w3331 -> [_ w3339]
                              tunnel: w3330 -> [_ w3338]
                              tunnel: w3329 -> [_ w3337]
                              tunnel: w3328 -> [_ w3336]
                              frame #0 {
                                n1772 = call "sub vi - defrag tdms v1.vi"("panel id"=w3335) -> ("error out"=w3334:errorcluster)  [unwired: 10 in]
                                n1773 = local write "data file error"(w3334) -> ()
                              }
                              frame #1 {
                                n1774 = Bundle("STATUS"=w3340, "OUT SERVER ADDRESS"=w3339, "FROM ACCOUNT"=w3338, "Mail Test File To:"=w3337, "Mail Test Fail"=w3336) -> (w3343:T26)  [unwired: 1 in]
                                n1775 = call "Save data file (pass-fail) v5.vi"("Input Cluster"=w3343, "panel id"=w3341) -> ("network file save error"=w3342:errorcluster)  [unwired: 8 in, 1 out]
                                n1776 = local write "data file error"(w3342) -> ()
                              }
                            }
                          }
                        }
                      }
                    }
                  }
                }
              }
            }
            n1777 = local read "Network Directory"() -> (w2857:path)
            n1778 = global write "Global 1.vi" "Network Drive"(w2857) -> ()
          }
          frame #8 {
            # "disable functions"
            n1779 = stacked-sequence {
              tunnel: w3353 -> [w3367 _ w3424]
              tunnel: w3352 -> [w3362 _ w3423]
